vi "Check Transmit Interval.vi"(6 "Local Data":T2 {"Last Transmit" format="%<%x %.3X>T"}, 7 "QRD":T1, 8 "error in":errorcluster) -> (0 "error out":errorcluster, 3 "Transmit Data?":bool, 4 "Local Data Out":T2 {"Last Transmit" format="%<%x %.3X>T"}, 5 "QRD Out":T1)   [LabVIEW 2025]
uses:
  Controls/Local Data_Acquisition.ctl
  Controls/Queues-Refs-Data.ctl
  Builds/Queue Wrappers.lvlibp/Q Packet.ctl
  Builds/Queue Wrappers.lvlibp
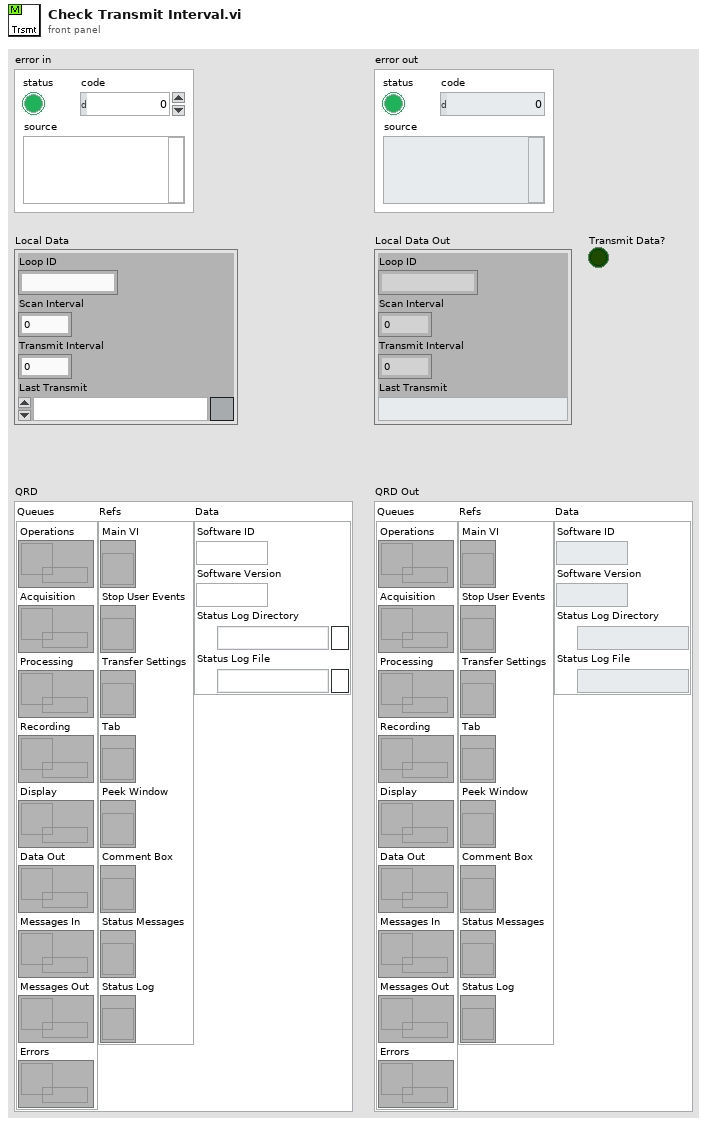
[diagram p1: front panel]
types:
  T1 = typedef "Queues-Refs-Data.ctl" = cluster{"Queues":cluster{"Operations":refnum<queue>, "Acquisition":refnum<queue>, "Processing":refnum<queue>, "Recording":refnum<queue>, "Display":refnum<queue>, "Data Out":refnum<queue>, "Messages In":refnum<queue>, "Messages Out":refnum<queue>, "Errors":refnum<queue>}, "Refs":cluster{"Main VI":refnum<vi>, "Stop User Events":refnum<vi>, "Transfer Settings":refnum<vi>, "Tab":refnum<vi>, "Peek Window":refnum<vi>, "Comment Box":refnum<vi>, "Status Messages":refnum<vi>, "Status Log":refnum<vi>}, "Data":cluster{"Software ID":string, "Software Version":string, "Status Log Directory":path, "Status Log File":path}}
  T2 = typedef "Local Data_Acquisition.ctl" = cluster{"Loop ID":string, "Scan Interval":u32, "Transmit Interval":u32, "Last Transmit":timestamp}
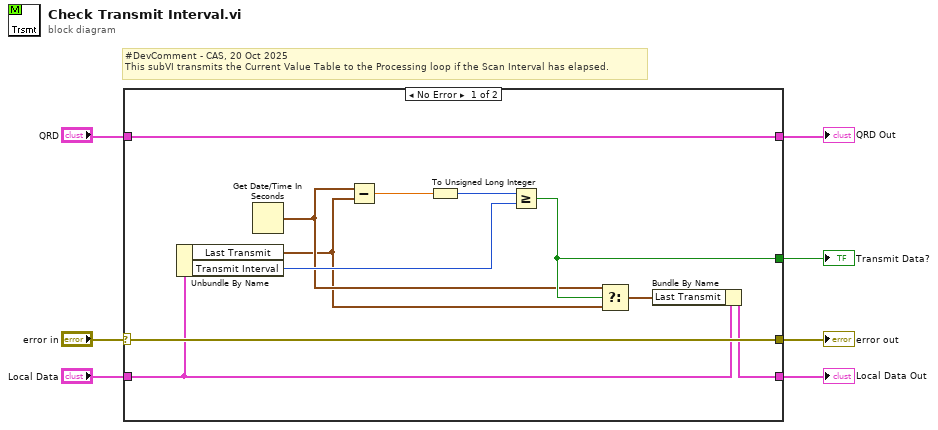
[diagram p0: block diagram]
diagram:
  # "#DevComment - CAS, 20 Oct 2025\nThis subVI transmits the Current Value Table to the Processing loop if the Scan Interval has elapsed."
  n1 = case shown="No Error" "error in" {
    selector: "error in" -> [w14 w19]
    tunnel: [w18 w21] -> w7
    tunnel: "QRD" -> [w18 w21]
    tunnel: [w13 w20] -> w5
    tunnel: "Local Data" -> [w12 w20]
    tunnel: [w14 w19] -> w3
    tunnel: [w10 _] -> w1
    frame No Error {
      n2 = Unbundle By Name(w12) -> ("Last Transmit"=w8:timestamp, "Transmit Interval"=w16:u32)
      n3 = Get Date/Time In Seconds() -> (seconds since 1Jan1904=w9:timestamp)
      n4 = Subtract(x=w9, y=w8) -> (x-y=w17:dbl)
      n5 = To Unsigned Long Integer(number=w17) -> (unsigned 32bit integer=w15:u32)
      n6 = Greater Or Equal?(x=w15, y=w16) -> (x >= y?=w10:bool)
      n7 = Select(t=w9, s=w10, f=w8) -> (s? t:f=w11:timestamp)
      n8 = Bundle By Name(cluster=w12, "Last Transmit"=w11) -> (w13:T2)
    }
    frame Error {
    }
  }
  "error out" <- w3
  "Local Data Out" <- w5
  "QRD Out" <- w7
  "Transmit Data?" <- w1
